vi "FuseTargeting.vi"(0 "Estimated Distance to Target (in)":dbl, 1 "Estimated Heading to Target (deg)":dbl, 7 "LIDAR Distance to Target (in)":dbl, 9 "LimeLight Distance to Target (in)":dbl, 11 "LimeLight Heading to Target (deg)":dbl, 13 "Robot_H (deg)":dbl) -> (14 "Fused Distance to Target (in)":dbl, 15 "Fused Heading to Target (deg)":dbl, 16 "Fused Heading to Target Delta (deg)":dbl, 17 "Pointed at Target":bool)   [LabVIEW 2019]
doc: "This VI fuses data from multiple sensing modalities to estimate the robot's range and heading-error to the target."
uses:
  dsdata.vi
  sensors.vi
panel:
  in  "Loops to Average Distance":i32=15
  in  "Min Timed Aligned (ms)":u32=200
  in  "Acceptable Heading Error (deg)":dbl=5.0
  in  "Loops to Average Heading":i32=15
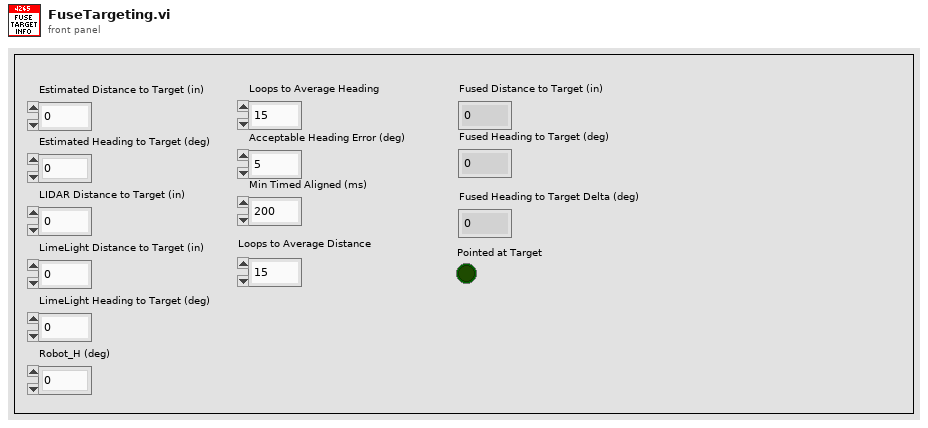
[diagram p1: front panel]
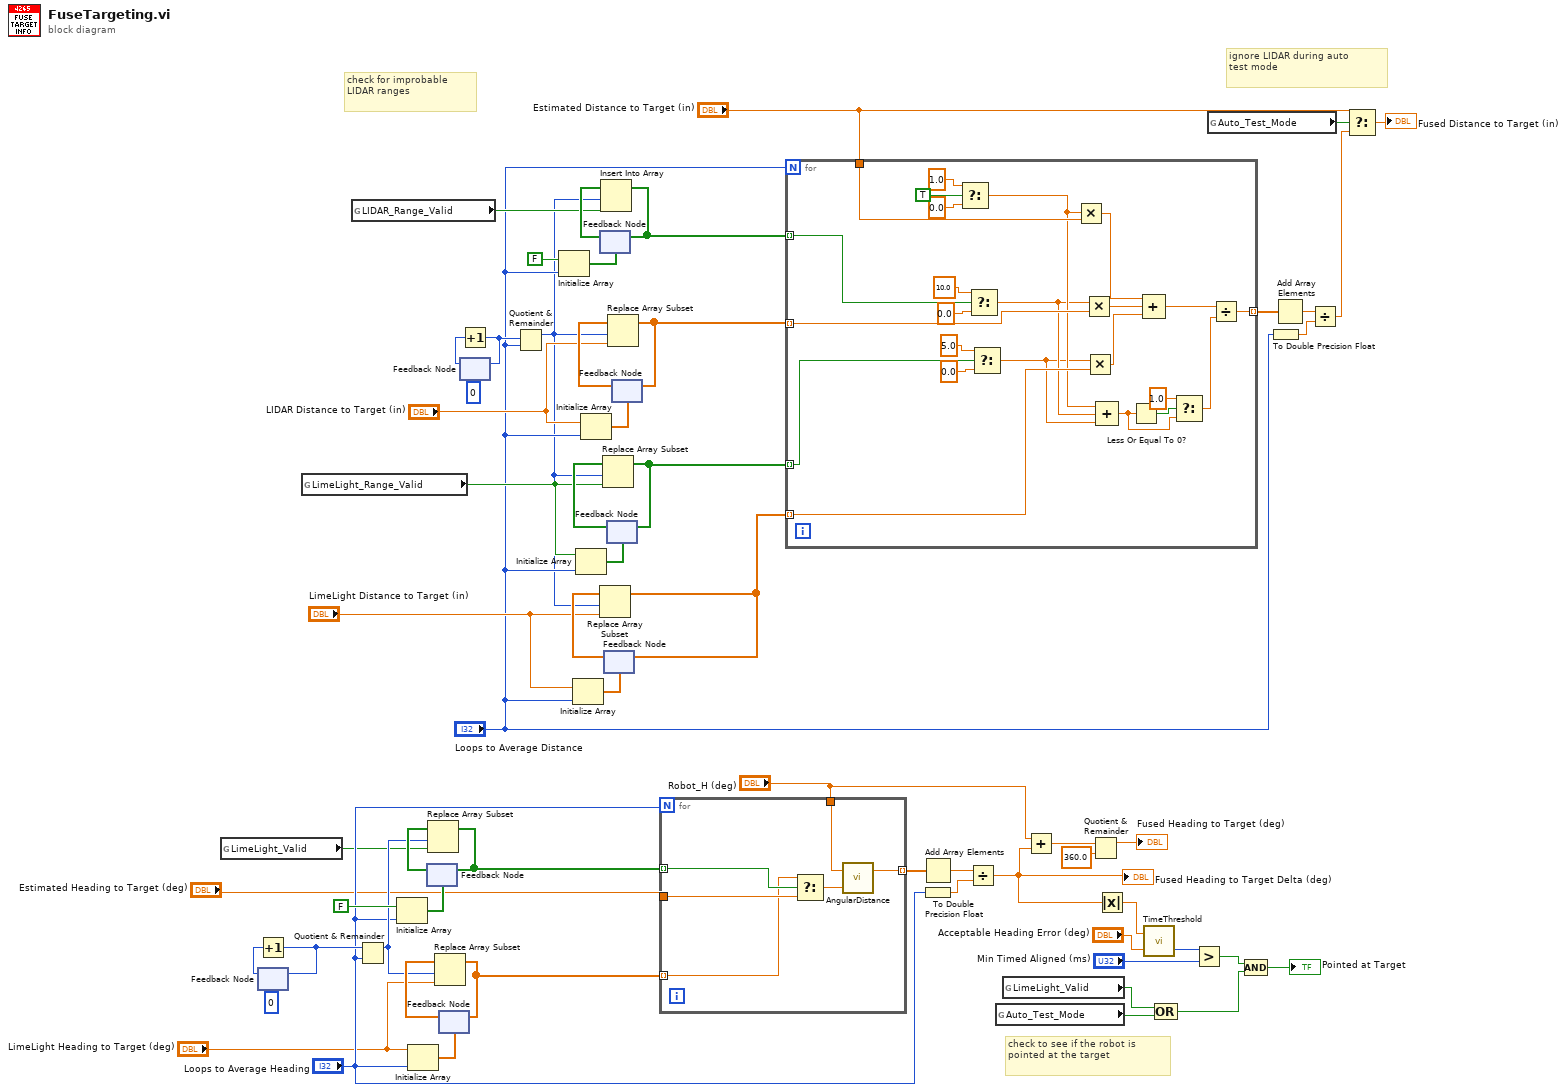
[diagram p0: block diagram]
diagram:
  # "check for improbable\nLIDAR ranges"
  # "check to see if the robot is\npointed at the target"
  # "ignore LIDAR during auto\ntest mode"
  n1 = global read "sensors.vi" "LimeLight_Valid"() -> (w23:bool)
  n2 = feedback #1(0) -> (w58:i32)
  n3 = Increment(x=w58) -> (x+1=w57:i32)
  n4 = feedback-in #1(w57) -> ()
  n5 = global read "sensors.vi" "LimeLight_Range_Valid"() -> (w13:bool)
  n6 = global read "sensors.vi" "LIDAR_Range_Valid"() -> (w16:bool)
  n7 = Quotient & Remainder(x=w57, y="Loops to Average Heading") -> (x-y*floor(x/y)=w52:i32)  [unwired: 1 out]
  n8 = Initialize Array(FALSE, "Loops to Average Heading") -> (w54:bool[])
  n9 = Initialize Array("LimeLight Heading to Target (deg)", "Loops to Average Heading") -> (w61:dbl[])
  n10 = feedback #2(w54) -> (w56:bool[])
  n11 = Replace Array Subset(array=w56, new element=w23, index=w52) -> (w53:bool[])
  n12 = feedback-in #2(w53) -> ()
  n13 = feedback #3(w61) -> (w60:dbl[])
  n14 = Replace Array Subset(array=w60, new element="LimeLight Heading to Target (deg)", index=w52) -> (w22:dbl[])
  n15 = feedback-in #3(w22) -> ()
  n16 = feedback #4(0) -> (w26:i32)
  n17 = Increment(x=w26) -> (x+1=w25:i32)
  n18 = feedback-in #4(w25) -> ()
  n19 = Quotient & Remainder(x=w25, y="Loops to Average Distance") -> (x-y*floor(x/y)=w7:i32)  [unwired: 1 out]
  n20 = Initialize Array(FALSE, "Loops to Average Distance") -> (w35:bool[])
  n21 = Initialize Array("LimeLight Distance to Target (in)", "Loops to Average Distance") -> (w10:dbl[])
  n22 = Initialize Array(w13, "Loops to Average Distance") -> (w15:bool[])
  n23 = Initialize Array("LIDAR Distance to Target (in)", "Loops to Average Distance") -> (w39:dbl[])
  n24 = feedback #5(w35) -> (w37:bool[])
  n25 = Insert Into Array(array=w37, index=w7, new element=w16) -> (w34:bool[])
  n26 = feedback-in #5(w34) -> ()
  n27 = feedback #6(w10) -> (w11:dbl[])
  n28 = Replace Array Subset(array=w11, new element="LimeLight Distance to Target (in)", index=w7) -> (w6:dbl[])
  n29 = feedback-in #6(w6) -> ()
  n30 = feedback #7(w15) -> (w14:bool[])
  n31 = Replace Array Subset(array=w14, new element=w13, index=w7) -> (w12:bool[])
  n32 = feedback-in #7(w12) -> ()
  n33 = feedback #8(w39) -> (w38:dbl[])
  n34 = Replace Array Subset(array=w38, new element="LIDAR Distance to Target (in)", index=w7) -> (w33:dbl[])
  n35 = feedback-in #8(w33) -> ()
  n36 = for {
    N: "Loops to Average Heading" -> [_]
    tunnel: w53 -> [w67] mode=indexing
    tunnel: w22 -> [w62] mode=indexing
    tunnel: "Estimated Heading to Target (deg)" -> [w66]
    tunnel: "Robot_H (deg)" -> [w65]
    tunnel: [w63] -> w51 mode=indexing
    n37 = Select(t=w62, s=w67, f=w66) -> (s? t:f=w64:dbl)
    n38 = call "AngularDistance.vi"("Goal Angle (deg) [0,360]"=w64, "Current Angle (deg) [-Inf,+Inf]"=w65) -> ("Signed Angular Distance (deg) [-180,+180]"=w63:dbl)  [unwired: 1 out]
  }
  n39 = for {
    N: "Loops to Average Distance" -> [_]
    tunnel: w34 -> [w78] mode=indexing
    tunnel: w33 -> [w79] mode=indexing
    tunnel: w12 -> [w77] mode=indexing
    tunnel: w6 -> [w76] mode=indexing
    tunnel: "Estimated Distance to Target (in)" -> [w80]
    tunnel: [w75] -> w4 mode=indexing
    n40 = Select(t=1.0, s=TRUE, f=0.0) -> (s? t:f=w74:dbl)
    n41 = Select(t=10.0, s=w78, f=0.0) -> (s? t:f=w73:dbl)
    n42 = Select(t=5.0, s=w77, f=0.0) -> (s? t:f=w72:dbl)
    n43 = Multiply(x=w74, y=w80) -> (x*y=w86:dbl)
    n44 = Multiply(x=w73, y=w79) -> (x*y=w85:dbl)
    n45 = Multiply(x=w72, y=w76) -> (x*y=w82:dbl)
    n46 = Compound Arithmetic op=ADD(w74, w73, w72) -> (w70:dbl)
    n47 = Less Or Equal To 0?(x=w70) -> (x <= 0?=w71:bool)
    n48 = Compound Arithmetic op=ADD(w86, w85, w82) -> (w91:dbl)
    n49 = Select(t=1.0, s=w71, f=w70) -> (s? t:f=w68:dbl)
    n50 = Divide(x=w91, y=w68) -> (x/y=w75:dbl)
  }
  n51 = Add Array Elements(numeric array=w51) -> (sum=w50:dbl)
  n52 = To Double Precision Float(number="Loops to Average Heading") -> (double precision float=w49:dbl)
  n53 = Divide(x=w50, y=w49) -> (x/y=w17:dbl)
  "Fused Heading to Target Delta (deg)" <- w17
  n54 = global read "dsdata.vi" "Auto_Test_Mode"() -> (w3:bool)
  n55 = global read "sensors.vi" "LimeLight_Valid"() -> (w2:bool)
  n56 = Add(x="Robot_H (deg)", y=w17) -> (x+y=w21:dbl)
  n57 = Quotient & Remainder(x=w21, y=360.0) -> (x-y*floor(x/y)=→"Fused Heading to Target (deg)":dbl)  [unwired: 1 out]
  n58 = Absolute Value(x=w17) -> (abs(x)=w44:dbl)
  n59 = call "TimeThreshold.vi"("Threshold"="Acceptable Heading Error (deg)", "Current Value"=w44) -> ("Time Below Threshold (ms)"=w42:u32)  [unwired: 1 out]
  n60 = Compound Arithmetic op=OR(w2, w3) -> (w1:bool)
  n61 = Greater?(x=w42, y="Min Timed Aligned (ms)") -> (0:w40:bool)
  n62 = global read "dsdata.vi" "Auto_Test_Mode"() -> (w45:bool)
  n63 = Compound Arithmetic op=AND(w40, w1) -> (→"Pointed at Target":bool)
  n64 = To Double Precision Float(number="Loops to Average Distance") -> (double precision float=w31:dbl)
  n65 = Add Array Elements(numeric array=w4) -> (sum=w32:dbl)
  n66 = Divide(x=w32, y=w31) -> (x/y=w30:dbl)
  n67 = Select(t="Estimated Distance to Target (in)", s=w45, f=w30) -> (s? t:f=→"Fused Distance to Target (in)":dbl)
